vi "Phasor User-defined Gate & IRF.vi"() -> ()   [LabVIEW 2021, in "Phasor.lvlib"]
uses:
  Graphs/XY Graph/XY Plot Data.ctl
  Phasor.lvlib
  Graphs/XY Graph/XY Graph Add-Ons.lvlib
panel:
  in  "User-defined IRF":T1
  in  "User-defined Gate":T1
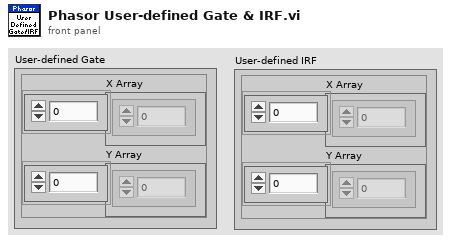
[diagram p1: front panel]
types:
  T1 = typedef "XY Graph Add-Ons.lvlib/XY Plot Data.ctl" = cluster{"X Array":dbl[], "Y Array":dbl[]}
diagram:
